vi "Example Simple.vi"() -> ()   [LabVIEW 2013]
uses:
  C:/tf/play/labview/Tinkerforge.dll
panel:
  out "logitude (°)":string
  out "latitude (°)":string
  in  "uid":string="ABC"
  in  "port":i32=4223
  in  "host":string="localhost"
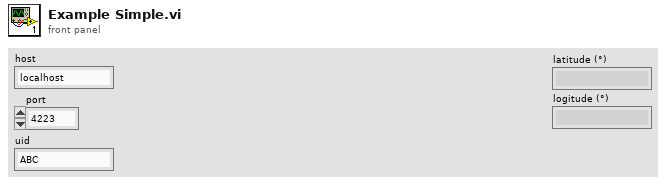
[diagram p1: front panel]
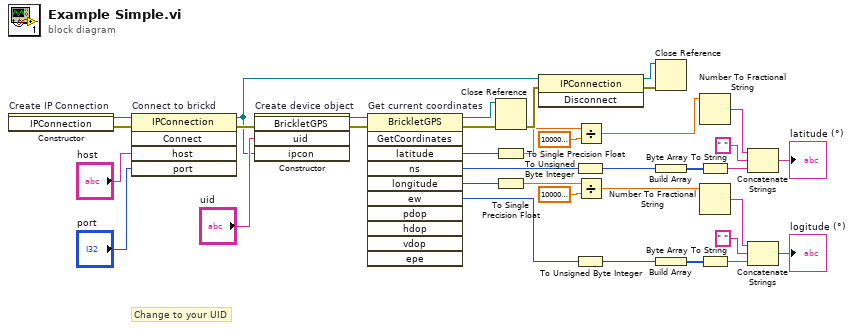
[diagram p0: block diagram]
diagram:
  # "Change to your UID"
  n1 = constructor on="Create IP Connection" class="IPConnection"() -> (reference out=w36:refnum<k24>, error out=w21:errorcluster)  [unwired: 3 in, 1 out]
  n2 = invoke on="Connect to brickd" class="IPConnection" method="Connect"(reference=w36, error in=w21, "host"="host", "port"="port") -> (reference out=w25:refnum<k24>, error out=w32:errorcluster)  [unwired: 1 in, 3 out]
  n3 = constructor on="Create device object" class="BrickletGPS"(error in=w32, "uid"="uid", "ipcon"=w25) -> (reference out=w30:refnum<k24>, error out=w31:errorcluster)  [unwired: 2 in, 3 out]
  n4 = invoke on="Get current coordinates" class="BrickletGPS" method="GetCoordinates"(reference=w30, error in=w31) -> (reference out=w28:refnum<k24>, error out=w29:errorcluster, "latitude"=w20:i64, "ns"=w17:u16, "longitude"=w4:i64, "ew"=w3:u16)  [unwired: 9 in, 5 out]
  n5 = Close Reference(reference=w28, error in (no error)=w29) -> (error out=w27:errorcluster)
  n6 = To Single Precision Float(number=w20) -> (single precision float=w23:sgl)
  n7 = To Single Precision Float(number=w4) -> (single precision float=w11:sgl)
  n8 = invoke class="IPConnection" method="Disconnect"(reference=w25, error in=w27) -> (reference out=w24:refnum<k24>, error out=w26:errorcluster)  [unwired: 1 in, 1 out]
  n9 = To Unsigned Byte Integer(number=w17) -> (unsigned 8bit integer=w16:u8)
  n10 = To Unsigned Byte Integer(number=w3) -> (unsigned 8bit integer=w8:u8)
  n11 = Divide(x=w23, y=sgl 1000000.0) -> (x/y=w19:sgl)
  n12 = Divide(x=w11, y=sgl 1000000.0) -> (x/y=w1:sgl)
  n13 = Close Reference(reference=w24, error in (no error)=w26) -> ()  [unwired: 1 out]
  n14 = Build Array(w16) -> (w18:u8[])
  n15 = Build Array(w8) -> (w9:u8[])
  n16 = Number To Fractional String(number=w19) -> (F-format string=w15:string)  [unwired: 3 in]
  n17 = Byte Array To String(unsigned byte array=w18) -> (string=w12:string)
  n18 = Number To Fractional String(number=w1) -> (F-format string=w2:string)  [unwired: 3 in]
  n19 = Byte Array To String(unsigned byte array=w9) -> (string=w5:string)
  n20 = Concatenate Strings(w15, " ", w12) -> (→"latitude (°)":string)
  n21 = Concatenate Strings(w2, " ", w5) -> (→"logitude (°)":string)
